vi "LF Write File (STR).vi"(4 "convert eol (F)":bool, 5 "data":string, 7 "error in (no error)":errorcluster, 8 "offset in (0)":dbl, 9 "pos mode (current)":enum16{"start", "end", "current"}(ring)=enum."current", 10 "refnum":refnum<file>) -> (0 "error out":errorcluster, 1 "offset out":dbl, 3 "refnum out":refnum<file>)   [LabVIEW 2009]
uses:
  kernel32.dll
panel:
  # "max offset is limited to about\n2^51 (1 000 000 000 000 000)  bytes\nto maintain full resolution of 1 bytes"
  # "LF Write File (STR).vi\n\nWrites an string using a double precision number as offset to work for files larger than 2GB.\n\nPlease visit http://www.OpenG.org to learn about the\nOpen Source LabVIEW software movement.\n\nNOTICE -- YOU MUST LEAVE THIS NOTICE IN PLACE.  PER THE TERMS OF THE LICENSE BELOW, YOU MAY SUBLICENSE THIS SOFTWARE \nIN ANY WAY THAT DOES NOT CONFLICT WITH THIS LICENSE.\n\n### BSD License (http://www.opensource.org/licenses/bsd-license.php) Begin ###\n\nCopyright (c) 2003, Rolf Kalbermatter <rolf.kalbermatter@citeng.com>\n\nAll rights reserved.\n\nRedistribution and use in source and binary forms, with or without modification, are permitted provided that the following conditions are met:\n\n    * Redistributions of source code must retain the above copyright notice, this list of conditions and the following disclaimer.\n    * Redistributions in binary form must reproduce the above copyright notice, this list of conditions and the following disclaimer in the \n       documentation and/or other materials provided with the distribution.\n    * Neither the name of SciWare, James Kring, Inc., nor the names of its contributors may be used to endorse or promote products derived \n       from this software without specific prior written permission.\n\nTHIS SOFTWARE IS PROVIDED BY THE COPYRIGHT HOLDERS AND CONTRIBUTORS \"AS IS\" AND ANY EXPRESS OR IMPLIED WARRANTIES, \nINCLUDING, BUT NOT LIMITED TO, THE IMPLIED WARRANTIES OF MERCHANTABILITY AND FITNESS FOR A PARTICULAR PURPOSE ARE \nDISCLAIMED. IN NO EVENT SHALL THE COPYRIGHT OWNER OR CONTRIBUTORS BE LIABLE FOR ANY DIRECT, INDIRECT, INCIDENTAL,\n SPECIAL, EXEMPLARY, OR CONSEQUENTIAL DAMAGES (INCLUDING, BUT NOT LIMITED TO, PROCUREMENT OF SUBSTITUTE GOODS OR \nSERVICES; LOSS OF USE, DATA, OR PROFITS; OR BUSINESS INTERRUPTION) HOWEVER CAUSED AND ON ANY THEORY OF LIABILITY, \nWHETHER IN CONTRACT, STRICT LIABILITY, OR TORT (INCLUDING NEGLIGENCE OR OTHERWISE) ARISING IN ANY WAY OUT OF THE USE \nOF THIS SOFTWARE, EVEN IF ADVISED OF THE POSSIBILITY OF SUCH DAMAGE.\n\n### BSD License End ###"
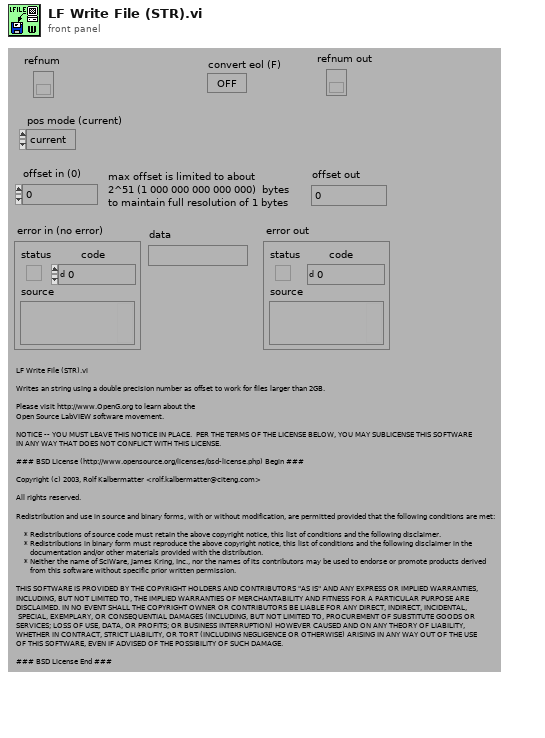
[diagram p1: front panel]
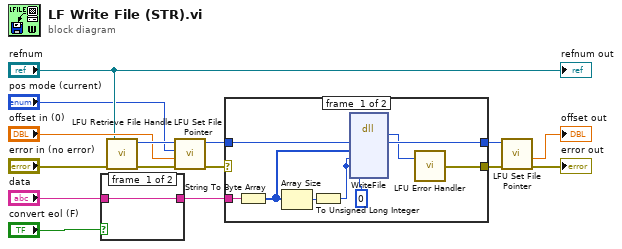
[diagram p0: block diagram]
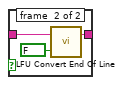
[diagram p2: hidden frame]
diagram:
  n1 = case shown="True" "convert eol (F)" {
    tunnel: "data" -> [w16 w19]
    tunnel: [w16 w18] -> w2
    frame #0 {
    }
    frame #1 {
      n2 = call "LFU Convert End Of Line.vi"("convert to LV"=FALSE, "input"=w19) -> ("output"=w18:string)  [unwired: 1 in]
    }
  }
  n3 = call "LFU Retrieve File Handle.vi"("error in (no error)"="error in (no error)", "file refnum"="refnum") -> ("error out"=w13:errorcluster, "handle out"=w14:u32)  [unwired: 4 in]
  n4 = call "LFU Set File Pointer.vi"("error in (no error)"=w13, "offset in (0)"="offset in (0)", "pos mode (current)"="pos mode (current)", "handle"=w14) -> ("error out"=w7:errorcluster, "handle out"=w6:u32)  [unwired: 1 in, 1 out]
  n5 = case shown="No Error" w7 {
    selector: w7 -> [_ w30]
    tunnel: w6 -> [w27 w29]
    tunnel: w2 -> [w26 _]
    tunnel: [w25 w29] -> w5
    tunnel: [w23 w30] -> w4
    frame #0 {
      n6 = String To Byte Array(string=w26) -> (unsigned byte array=w20:u8[])
      n7 = Array Size(array=w20) -> (size(s)=w24:i32)
      n8 = To Unsigned Long Integer(number=w24) -> (unsigned 32bit integer=w21:u32)
      n9 = dll-call lib="kernel32.dll" fn="WriteFile"("handle"=w27, "buffer"=w20, "bytesToRead"=w21, "bytesRead"=w21, "overlapped"=u32 0) -> (w22:u32, "handle"=w25:u32)  [unwired: 7 in, 2 out]
      n10 = call "LFU Error Handler.vi"("retval"=w22) -> ("error out"=w23:errorcluster)  [unwired: 1 in]
    }
    frame #1 {
    }
  }
  n11 = call "LFU Set File Pointer.vi"("error in (no error)"=w4, "handle"=w5) -> ("error out"=→"error out":errorcluster, "offset out"=→"offset out":dbl)  [unwired: 3 in, 1 out]
  "refnum out" <- "refnum"
